vi "CMD_HOME.vi"(9 "Chan Ident":string="1") -> (1 "Command":string)   [LabVIEW 2017]
panel:
  out "x = y?":bool
  in  "ReqCmd 2":string="D\u0004040600A2010100400D0300"
  # "CMD_ABS_POS"
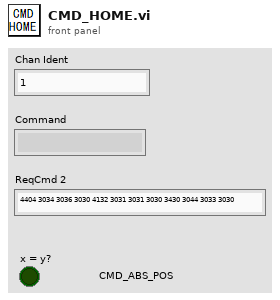
[diagram p1: front panel]
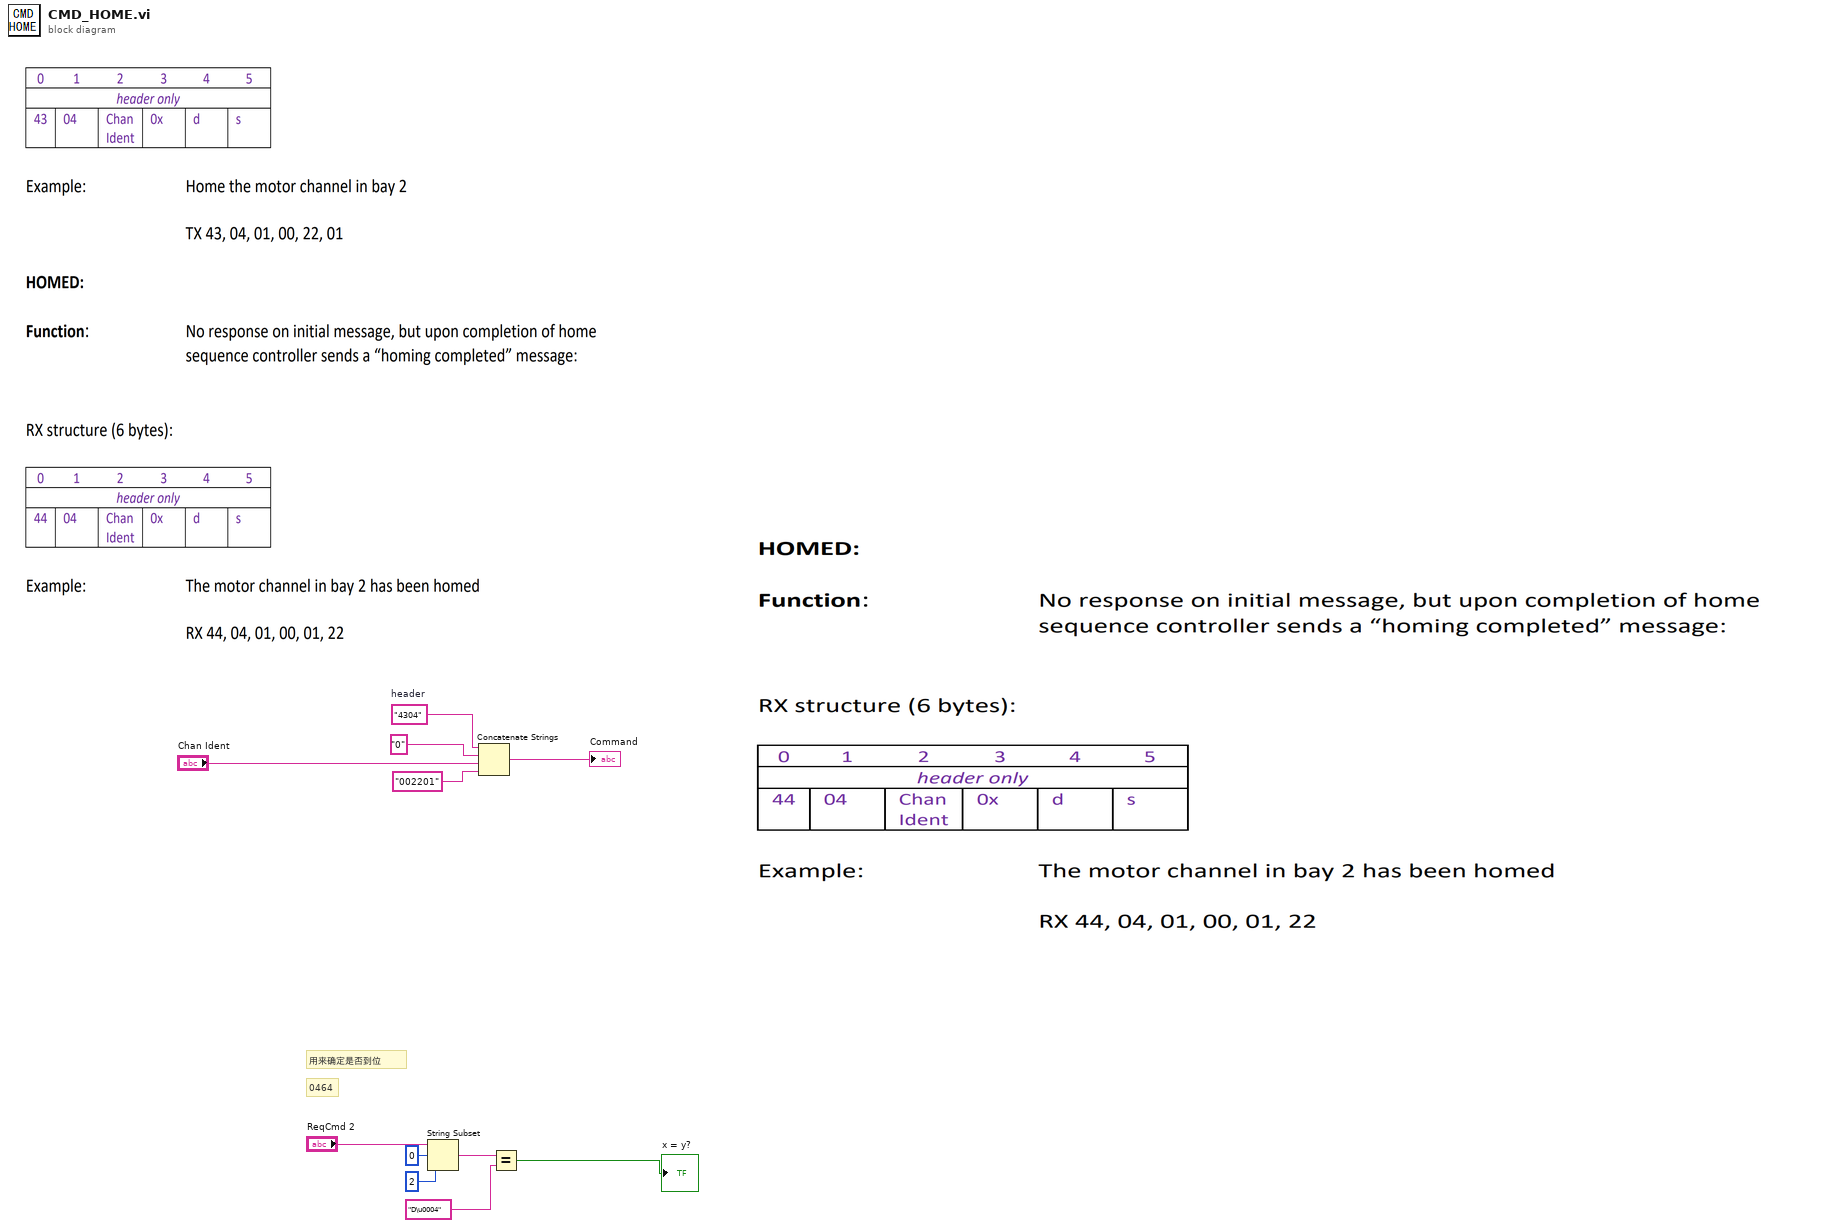
[diagram p0: block diagram]
diagram:
  w9 = "4304"  # header
  # "用来确定是否到位"
  # "0464"
  n1 = String Subset(string="ReqCmd 2", offset (0)=0 ("偏移量(0)"), length (rest)=2 ("长度（剩余）")) -> (substring=w3:string)
  n2 = Concatenate Strings(w9, "0" ("字符串"), "Chan Ident", "002201" ("字符串")) -> (→"Command":string)
  n3 = Equal?(x=w3, y="D\u0004") -> (x = y?=→"x = y?":bool)
